vi "Desired Arm Position.vi"() -> ()   [LabVIEW 2014]
panel:
  in  "Desired Back Arm Speed":dbl
  in  "Desired Front Arm Position":dbl
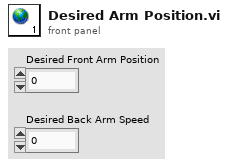
[diagram p1: front panel]
diagram:
